vi "Panel-BC.vi"() -> ()   [LabVIEW 2009]
uses:
  Instruments/Motor/Controls/MotorStatus.ctl
panel:
  out "BC-FIP2-Z":T1
  out "BC-FIP1-Z":T1
  in  "BC-FIP2-X,BC-FIP2-Y":bool
  in  "BC-FIP1-X,BC-FIP1-Y":bool
  out "BC-FIP2-Y":T1
  out "BC-FIP2-X":T1
  in  "stop":bool
  out "BC-FIP1-Y":T1
  out "BC-FIP1-X":T1
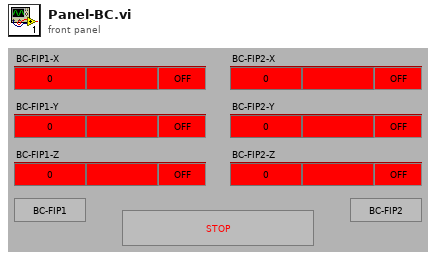
[diagram p1: front panel]
types:
  T1 = typedef "MotorStatus.ctl" = cluster{"Managed?":bool, "Position":i32, "Name":string, "Status":enum16{"OFF", "IDLE", "MOVING", "HOMING"}}
  T2 = enum32{"Invalid", "Standard", "Closed", "Hidden", "Minimized", "Maximized"}
  T3 = enum32{"Bad", "Idle", "Run top level", "Running"}
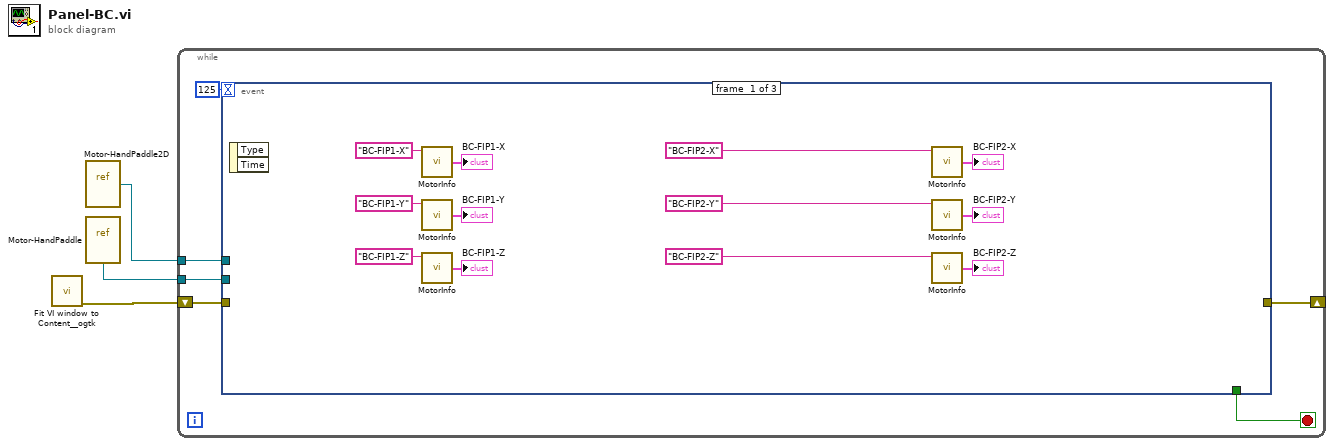
[diagram p0: block diagram]
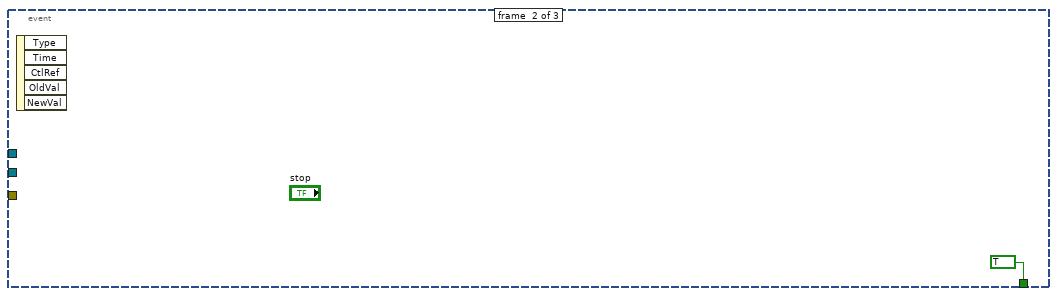
[diagram p2: hidden frame]
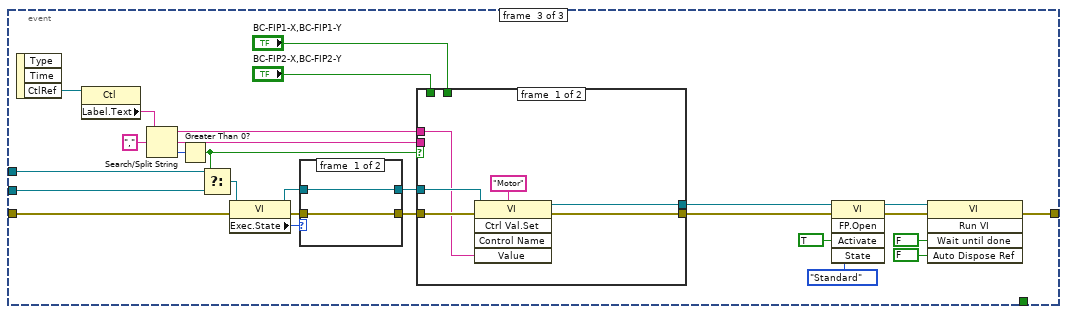
[diagram p3: hidden frame]
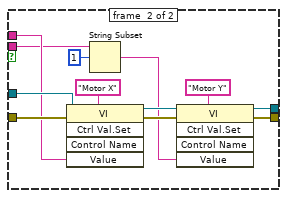
[diagram p4: hidden frame]
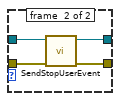
[diagram p5: hidden frame]
diagram:
  n1 = call <userlib>:"Fit VI window to Content__ogtk.vi"() -> ("error out"=w2:errorcluster)  [unwired: 6 in, 1 out]
  n2 = vi-ref "Motor-HandPaddle2D.vi"() -> (w1:refnum<vi>)
  n3 = vi-ref "Motor-HandPaddle.vi"() -> (w3:refnum<vi>)
  n4 = while {
    shift-right: [w7] -> _
    shift-left: w2 -> [w6]
    tunnel: w3 -> [w5]
    tunnel: w1 -> [w4]
    stop <- w8 stop-if-true
    n5 = event shown="[2] \"BC-FIP1-X\", \"BC-FIP1-Y\", \"BC-FIP2-X\", \"BC-FIP2-Y\", \"BC-FIP1-Z\", \"BC-FIP2-Z\": Mouse Down;  \"BC-FIP1-X,BC-FIP1-Y\", \"BC-FIP2-X,BC-FIP2-Y\": Value Change" {
      selector: _ -> [_ _ _]
      dyn-events: _ -> [_ _ _]
      timeout: 125 -> [_ _ _]
      tunnel: [_ TRUE _] -> w8
      tunnel: w6 -> [_ _ w36]
      tunnel: [_ _ w35] -> w7
      tunnel: w5 -> [_ _ w30]
      tunnel: w4 -> [_ _ w32]
      event #0 {
        n6 = event-data() -> ()  [unwired: 1 in, 2 out]
        n7 = call "MotorInfo.vi"("Motor"="BC-FIP1-X") -> ("Axis status"=→"BC-FIP1-X":T1)  [unwired: 1 in, 7 out]
        n8 = call "MotorInfo.vi"("Motor"="BC-FIP1-Y") -> ("Axis status"=→"BC-FIP1-Y":T1)  [unwired: 1 in, 7 out]
        n9 = call "MotorInfo.vi"("Motor"="BC-FIP1-Z") -> ("Axis status"=→"BC-FIP1-Z":T1)  [unwired: 1 in, 7 out]
        n10 = call "MotorInfo.vi"("Motor"="BC-FIP2-X") -> ("Axis status"=→"BC-FIP2-X":T1)  [unwired: 1 in, 7 out]
        n11 = call "MotorInfo.vi"("Motor"="BC-FIP2-Y") -> ("Axis status"=→"BC-FIP2-Y":T1)  [unwired: 1 in, 7 out]
        n12 = call "MotorInfo.vi"("Motor"="BC-FIP2-Z") -> ("Axis status"=→"BC-FIP2-Z":T1)  [unwired: 1 in, 7 out]
      }
      event #1 {
        n13 = event-data() -> ()  [unwired: 1 in, 5 out]
      }
      event #2 {
        n14 = event-data() -> ("CtlRef"=w34:refnum<vi>)  [unwired: 1 in, 2 out]
        n15 = property class="Ctl"(reference=w34) -> ("Label.Text"=w29:string)  [unwired: 1 in, 2 out]
        n16 = Search/Split String(string=w29, search string/char (-)=",") -> (substring before match=w26:string, match + rest of string=w28:string, offset of match=w27:i32)  [unwired: 1 in]
        n17 = Greater Than 0?(x=w27) -> (x > 0?=w25:bool)
        n18 = Select(t=w32, s=w25, f=w30) -> (s? t:f=w31:refnum<vi>)
        n19 = property class="VI"(reference=w31, error in=w36) -> (reference out=w38:refnum<vi>, error out=w39:errorcluster, "Exec.State"=w41:T3)
        n20 = case shown="\"Run top level\", \"Running\"" w41 {
          tunnel: w38 -> [w68 w72]
          tunnel: [w68 w69] -> w37
          tunnel: [w67 w70] -> w40
          tunnel: w39 -> [w67 w71]
          frame #0 {
          }
          frame #1 {
            n21 = call "SendStopUserEvent.vi"("VI Refnum in"=w72, "error in"=w71) -> ("VI Refnum out"=w69:refnum<vi>, "error out"=w70:errorcluster)  [unwired: 6 out]
          }
        }
        n22 = case shown="True" w25 {
          tunnel: [w55 w66] -> w47
          tunnel: [w54 w60] -> w42
          tunnel: w40 -> [w53 w65]
          tunnel: w37 -> [w52 w64]
          tunnel: w28 -> [_ w58]
          tunnel: w26 -> [w50 w59]
          tunnel: "BC-FIP1-X,BC-FIP1-Y" -> [_ _]
          tunnel: "BC-FIP2-X,BC-FIP2-Y" -> [_ _]
          frame #0 {
            n23 = invoke class="VI" method="Ctrl Val.Set"(reference=w52, error in=w53, "Control Name"="Motor", "Value"=w50) -> (reference out=w54:refnum<vi>, error out=w55:errorcluster)  [unwired: 1 in, 3 out]
          }
          frame #1 {
            n24 = invoke class="VI" method="Ctrl Val.Set"(reference=w64, error in=w65, "Control Name"="Motor X", "Value"=w59) -> (reference out=w61:refnum<vi>, error out=w66:errorcluster)  [unwired: 1 in, 3 out]
            n25 = String Subset(string=w58, offset (0)=1) -> (substring=w56:string)  [unwired: 1 in]
            n26 = invoke class="VI" method="Ctrl Val.Set"(reference=w61, "Control Name"="Motor Y", "Value"=w56) -> (reference out=w60:refnum<vi>)  [unwired: 2 in, 4 out]
          }
        }
        n27 = invoke class="VI" method="FP.Open"(reference=w42, error in=w47, "Activate"=TRUE ("Activate?"), "State"=T2."Standard") -> (reference out=w45:refnum<vi>, error out=w46:errorcluster)  [unwired: 1 in, 3 out]
        n28 = invoke class="VI" method="Run VI"(reference=w45, error in=w46, "Wait until done"=FALSE ("Wait Until Done"), "Auto Dispose Ref"=FALSE ("Auto Dispose Reference")) -> (error out=w35:errorcluster)  [unwired: 1 in, 4 out]
      }
    }
  }
